vi "Cluster Dialog_Double Click OK.vi"(9 "PlatMods":T1, 10 "Coords":cluster{"Horizontal":i32, "Vertical":i32}, 11 "TreeControl in":refnum<vi>) -> (3 "Valid Item Double Clicked":bool)   [LabVIEW 2023]
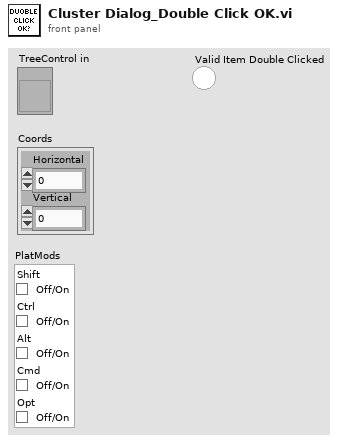
[diagram p1: front panel]
types:
  T1 = cluster{"Shift":bool, "Ctrl":bool, "Alt":bool, "Cmd":bool, "Opt":bool}
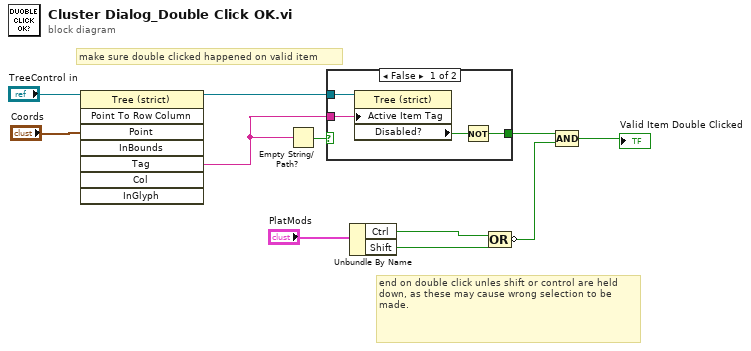
[diagram p0: block diagram]
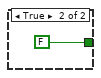
[diagram p2: hidden frame]
diagram:
  # "make sure double clicked happened on valid item"
  # "end on double click unles shift or control are held down, as these may cause wrong selection to be made."
  n1 = invoke class="Tree (strict)" method="Point To Row Column"(reference="TreeControl in", "Point"="Coords") -> (reference out=w4:refnum<vi>, "Tag"=w2:string)  [unwired: 6 in, 6 out]
  n2 = Empty String/Path?(string/path=w2) -> (empty?=w1:bool)
  n3 = case shown="False" w1 {
    tunnel: w4 -> [w15 _]
    tunnel: [w12 FALSE ("Disabled?")] -> w3
    tunnel: w2 -> [w13 _]
    frame False {
      n4 = property class="Tree (strict)"(reference=w15, "Active Item Tag"=w13) -> ("Disabled?"=w14:bool)  [unwired: 1 in, 2 out]
      n5 = Not(x=w14) -> (.not. x?=w12:bool)
    }
    frame True {
    }
  }
  n6 = Unbundle By Name("PlatMods") -> ("Ctrl"=w8:bool, "Shift"=w7:bool)
  n7 = Compound Arithmetic op=OR(w8, w7) -> (invert w6:bool)
  n8 = Compound Arithmetic op=AND(w3, w6) -> (→"Valid Item Double Clicked":bool)
